vi "S2DS- External Write-IPS current.vi"() -> ()   [LabVIEW 2016]
doc: "Uses DataSocket to read array data. \n \nThe Writer, Server, and Reader can all be on the same computer or different computers. The Writer and Reader URLs should point to the computer where the DataSocket Server is."
uses:
  source/TYPE DEFS/S2DS_Instrument parameters.ctl
panel:
  in  "Instrument parameters":T1
  in  "Sweep rate (A/min)":dbl
  in  "External":bool
  in  "Set Current (A)":dbl
  in  "Stop":bool
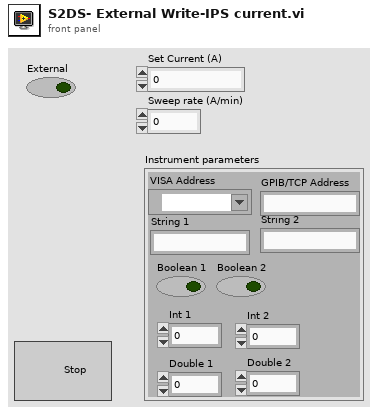
[diagram p1: front panel]
types:
  T1 = typedef "S2DS_Instrument parameters.ctl" = cluster{"VISA Address":refnum<visa-resource-name>, "GPIB/TCP Address":string, "String 1":string, "String 2":string, "Boolean 1":bool, "Boolean 2":bool, "Int 1":i32, "Int 2":i32, "Double 1":dbl, "Double 2":dbl}
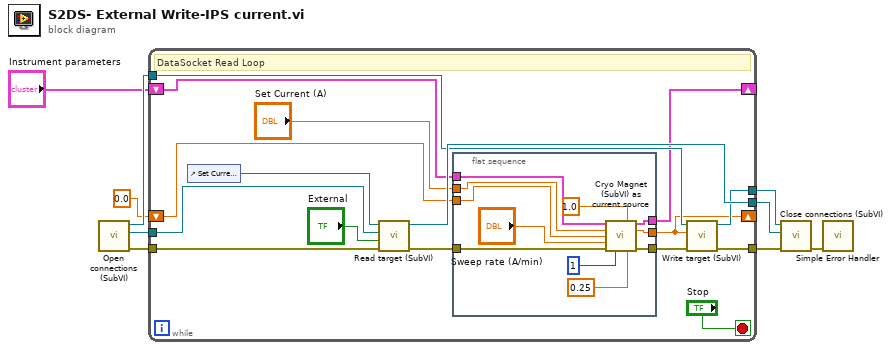
[diagram p0: block diagram]
diagram:
  n1 = call "Open connections (SubVI).vi"() -> ("error out"=w6:errorcluster, "Read connection"=w7:refnum<k13>, "Write connection"=w5:refnum<k13>)  [unwired: 9 in]
  n2 = while {
    tunnel: [w21] -> w9
    tunnel: w6 -> [w24]
    tunnel: w7 -> [w25]
    tunnel: [w23] -> w8
    tunnel: w5 -> [w22]
    tunnel: [w20] -> w4
    shift-right: [w12] -> _
    shift-left: 0.0 ("Last field") -> [w13]
    shift-right: [w10] -> _
    shift-left: "Instrument parameters" -> [w11]
    stop <- "Stop" stop-if-true
    # "DataSocket Read Loop"
    n3 = control-ref of="Set Current (A)"() -> (w17:refnum<vi>)
    n4 = call "Read target (SubVI).vi"("error in (no error)"=w24, "External"="External", "Read connection in"=w25, "Digital in"=w17) -> ("error out"=w14:errorcluster, "DataSocket Refnum out"=w23:refnum<k13>)  [unwired: 6 in]
    n5 = flat-sequence {
      tunnel: "Set Current (A)" -> [w36]
      tunnel: [w35] -> w12
      tunnel: [w31] -> w15
      tunnel: w14 -> [w32]
      tunnel: w13 -> [w34]
      tunnel: w11 -> [w30]
      tunnel: [w29] -> w10
      frame #0 {
        n6 = call "Cryo Magnet (SubVI) as current source.vi"("Instrument parameters"=w30, "Max Rate"=1.0, "Target"=w36, "Present value"=w34, "Sweep rate"="Sweep rate (A/min)", "error in (no error)"=w32, "Timeout (s)"=u16 1, "Default Rate"=0.25) -> ("Instrument parameters out"=w29:T1, "Last field"=w35:dbl, "error out"=w31:errorcluster)  [unwired: 5 in]
      }
    }
    n7 = call "Write target (SubVI).vi"("error in (no error)"=w15, "data to write"=w12, "DataSocket Refnum in"=w22) -> ("error out"=w21:errorcluster, "DataSocket Refnum out"=w20:refnum<k13>)  [unwired: 7 in]
  }
  n8 = call "Close connections (SubVI).vi"("error in (no error)"=w9, "Read connection"=w8, "Write connection"=w4) -> ("error out"=w3:errorcluster)  [unwired: 8 in]
  n9 = call <vilib>:"Simple Error Handler.vi"("error in (no error)"=w3) -> ()  [unwired: 4 in, 5 out]
